vi "RSZVB Get Mixer Delay Upper Tone Source.vi"(8 "error in (no error)":errorcluster {"code" format="%.0x"}, 10 "Channel (1)":i32=1, 11 "VISA session":refnum<visa-resource-name>) -> (0 "error out":errorcluster {"code" format="%.0x"}, 1 "Port number":i32, 2 "Source (1)":i32(ring)=1 items=["None", "Port", "Generator"], 3 "dup VISA session":refnum<visa-resource-name>)   [LabVIEW 2011]
doc: "Returns the source for the upper tone signal that is used for the mixer delay measurement.\n\nNotes:\n\n(1) This VI requires options R&S ZVA-K9 and R&S ZVA-K4.\n\nRemote-control command(s):\n[SENSe<Ch>:]FREQuency:MDELay:UTONe? PORT | GENerator"
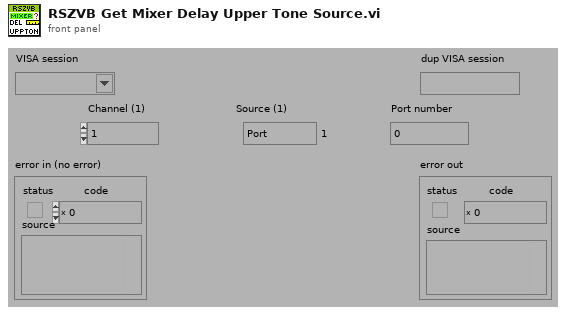
[diagram p1: front panel]
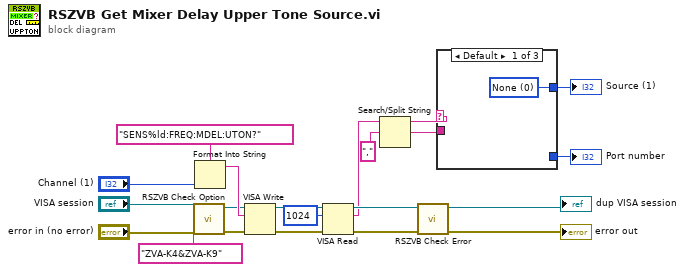
[diagram p0: block diagram]
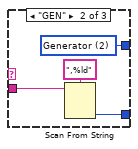
[diagram p2: hidden frame]
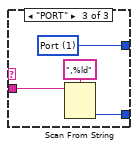
[diagram p3: hidden frame]
diagram:
  n1 = call "RSZVB Check Option.vi"("error in (no error)"="error in (no error)", "Options"="ZVA-K4&ZVA-K9", "VISA session"="VISA session") -> ("error out"=w7:errorcluster, "dup VISA session"=w8:refnum<visa-resource-name>)  [unwired: 7 in]
  n2 = Format Into String(format string="SENS%ld:FREQ:MDEL:UTON?", "Channel (1)") -> (resulting string=w16:string)  [unwired: 2 in, 1 out]
  n3 = VISA Write(VISA resource name=w8, write buffer=w16, error in (no error)=w7) -> (VISA resource name out=w14:refnum<visa-resource-name>, error out=w15:errorcluster)  [unwired: 1 out]
  n4 = VISA Read(VISA resource name=w14, byte count=u32 1024, error in (no error)=w15) -> (VISA resource name out=w11:refnum<visa-resource-name>, read buffer=w6:string, error out=w12:errorcluster)  [unwired: 1 out]
  n5 = Search/Split String(string=w6, search string/char (-)=",") -> (substring before match=w2:string, match + rest of string=w4:string)  [unwired: 1 in, 1 out]
  n6 = call "RSZVB Check Error.vi"("error in (no error)"=w12, "VISA session"=w11) -> ("error out"=→"error out":errorcluster, "dup VISA session"=→"dup VISA session":refnum<visa-resource-name>)  [unwired: 8 in]
  n7 = case shown="Default" w2 {
    tunnel: w4 -> [_ w25 w29]
    tunnel: [_ w24 w28] -> w3
    tunnel: [w22 w23 w27] -> w1
    frame Default {
      w22 = 0 items=["None", "Port", "Generator"] ("Source (1)")
    }
    frame "GEN" {
      w23 = 2 items=["None", "Port", "Generator"] ("Source (1)")
      n8 = Scan From String(format string=",%ld", input string=w25) -> (output 1=w24:i32)  [unwired: 3 in, 3 out]
    }
    frame "PORT" {
      w27 = 1 items=["None", "Port", "Generator"] ("Source (1)")
      n9 = Scan From String(format string=",%ld", input string=w29) -> (output 1=w28:i32)  [unwired: 3 in, 3 out]
    }
  }
  "Source (1)" <- w1
  "Port number" <- w3
